vi "Day 9-Compute Basin Sizes.vi"(10 "Padded Data Array in":i32[][](array[numeric]), 11 "Low Point Coordinates":i32[][](array[numeric])) -> (3 "All Basin Sizes":i32[](array[numeric]))   [LabVIEW 2021]
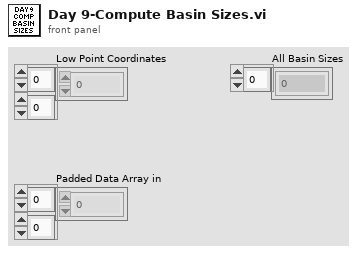
[diagram p1: front panel]
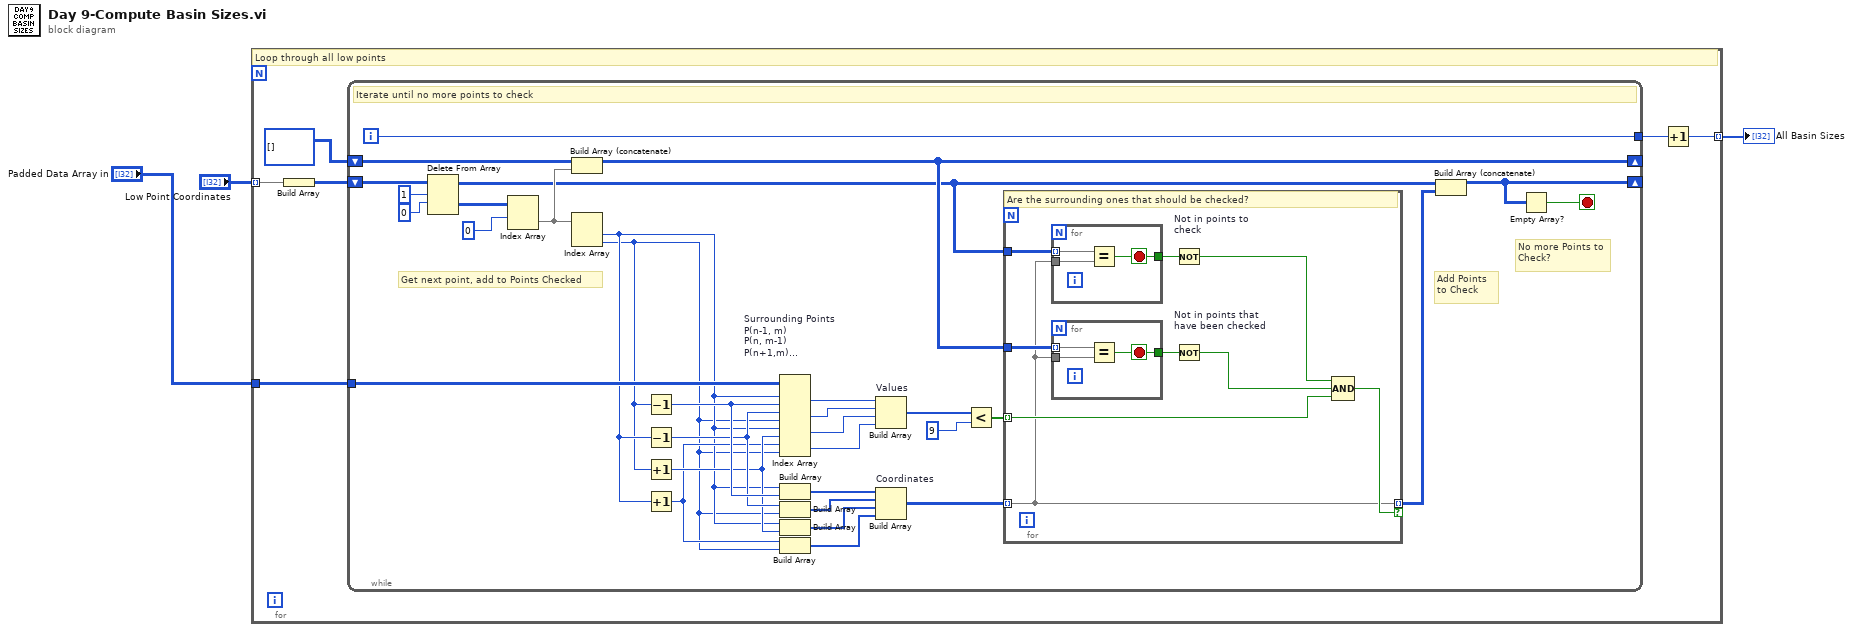
[diagram p0: block diagram]
diagram:
  n1 = for {
    tunnel: "Low Point Coordinates" -> [w9] mode=indexing
    tunnel: [w5] -> w1 mode=indexing
    tunnel: "Padded Data Array in" -> [w4]
    # "Loop through all low points"
    n2 = Build Array(w9) -> (w8:i32[][])
    n3 = while {
      shift-right: [w16] -> _
      shift-left: w8 -> [w24]
      tunnel: w4 -> [w41]
      tunnel: [w14] -> w7
      shift-right: [w11] -> _
      shift-left: i32[][] [] -> [w12]
      i -> [w14]
      stop <- w15 stop-if-true
      # "Get next point, add to Points Checked"
      # "No more Points to Check?"
      # "Add Points to Check"
      # "Iterate until no more points to check"
      n4 = Delete From Array(array=w24, length=1, index (row)=0) -> (deleted portion=w21:i32[][], array with subset deleted=w10:i32[][])  [unwired: 1 in]
      n5 = Index Array(array=w21, index (row)=0) -> (element=w13:i32[])  [unwired: 1 in]
      n6 = Build Array (concatenate)(w12, w13) -> (w11:i32[][])
      n7 = Index Array(array=w13) -> (element #1=w19:i32, element #2=w18:i32)  [unwired: 2 in]
      n8 = Decrement(x=w18) -> (x-1=w34:i32)
      n9 = Decrement(x=w19) -> (x-1=w33:i32)
      n10 = Increment(x=w18) -> (x+1=w32:i32)
      n11 = Increment(x=w19) -> (x+1=w31:i32)
      n12 = Index Array "Surrounding Points\nP(n-1, m)\nP(n, m-1)\nP(n+1,m)\nP(n, m+1)"(array=w41, index (row) #1=w19, index (col) #1=w34, index (row) #2=w33, index (col) #2=w18, index (row) #3=w19, index (col) #3=w32, index (row) #4=w31, index (col) #4=w18) -> (element #1=w40:i32, element #2=w39:i32, element #3=w38:i32, element #4=w37:i32)
      n13 = Build Array(w19, w34) -> (w30:i32[])
      n14 = Build Array(w33, w18) -> (w29:i32[])
      n15 = Build Array(w19, w32) -> (w28:i32[])
      n16 = Build Array(w31, w18) -> (w27:i32[])
      n17 = Build Array "Values"(w40, w39, w38, w37) -> (w36:i32[])
      n18 = Build Array "Coordinates"(w30, w29, w28, w27) -> (w25:i32[][])
      n19 = Less?(x=w36, y=9) -> (x < y?=w26:bool[])
      n20 = for {
        tunnel: w26 -> [w46] mode=indexing
        tunnel: w25 -> [w44] mode=indexing
        tunnel: [w44] -> w17 mode=indexing if=w47
        tunnel: w11 -> [w50]
        tunnel: w10 -> [w45]
        # "Are the surrounding ones that should be checked?"
        n21 = for {
          tunnel: w45 -> [w53] mode=indexing
          tunnel: w44 -> [w52]
          tunnel: [w51] -> w43
          stop <- w51 stop-if-true
          n22 = Equal?(x=w53, y=w52) -> (x = y?=w51:bool)
        }
        n23 = for {
          tunnel: w50 -> [w56] mode=indexing
          tunnel: w44 -> [w55]
          tunnel: [w54] -> w49
          stop <- w54 stop-if-true
          n24 = Equal?(x=w56, y=w55) -> (x = y?=w54:bool)
        }
        n25 = Not "Not in points to\ncheck"(x=w43) -> (.not. x?=w42:bool)
        n26 = Not "Not in points that\nhave been checked"(x=w49) -> (.not. x?=w48:bool)
        n27 = Compound Arithmetic op=AND(w42, w48, w46) -> (w47:bool)
      }
      n28 = Build Array (concatenate)(w10, w17) -> (w16:i32[][])
      n29 = Empty Array?(array=w16) -> (empty?=w15:bool)
    }
    n30 = Increment(x=w7) -> (x+1=w5:i32)
  }
  "All Basin Sizes" <- w1
